vi "ACC_LabVIEW_Connect.vi"(1 "Nomenklatur":string, 3 "return error strings buffer size (Byte)":u32=500, 5 "error in (no error)":errorcluster) -> (14 "DeviceReferenceOut":cluster{"ID":u32}, 19 "error out":errorcluster)   [LabVIEW 2014, in "ACC_LabVIEW.lvlib"]
doc: "Perform a \"read\" inside the GSI - accelerator control system."
uses:
  ACC_LabVIEW.lvlib
  lib/ACC_Interface_Wrapper.dll
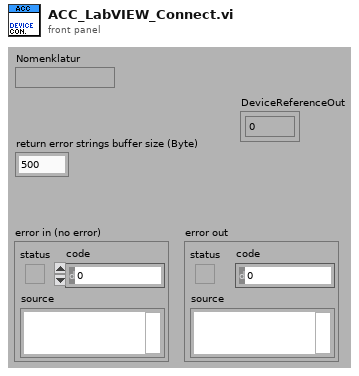
[diagram p1: front panel]
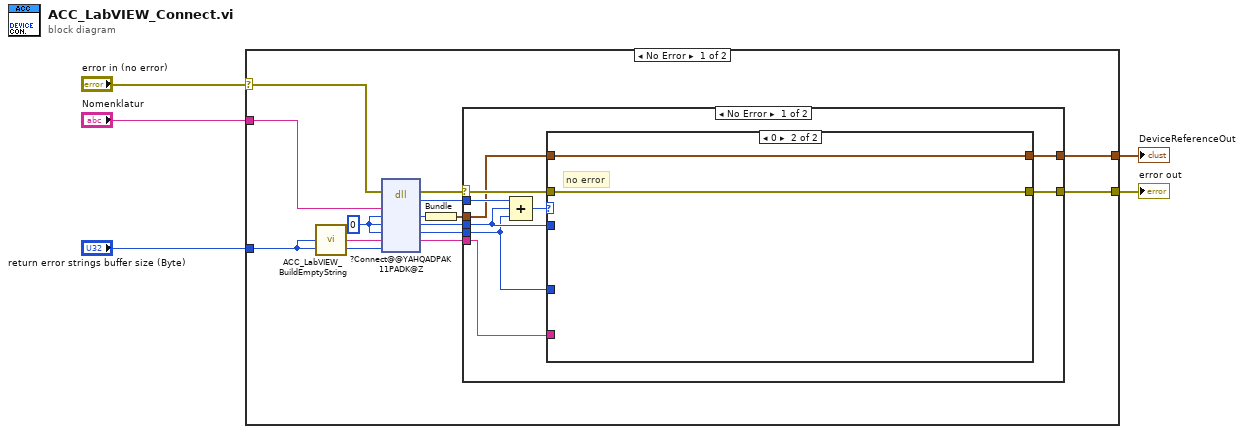
[diagram p0: block diagram]
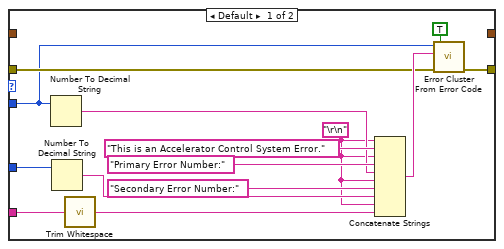
[diagram p2: hidden frame]
diagram:
  n1 = case shown="No Error" "error in (no error)" {
    selector: "error in (no error)" -> [w17 w46]
    tunnel: "Nomenklatur" -> [w18 _]
    tunnel: "return error strings buffer size (Byte)" -> [w15 _]
    tunnel: [w19 w46] -> w3
    tunnel: [w8 _] -> w1
    frame No Error {
      w9 = u32 0 ("no input, only output")
      n2 = call "ACC_LabVIEW_BuildEmptyString.vi"("Length"=w15) -> ("String"=w16:string)
      n3 = dll-call lib="D:/Git/CS-framework/CSinstr.lib/ACC_LabVIEW_Interface/lib/ACC_Interface_Wrapper.dll" fn="?Connect@@YAHQADPAK11PADK@Z"(error in=w17, "LV_nomenklatur"=w18, "DeviceHandle"=w9, "ErrPrimStat"=w9, "ErrSecStat"=w9, "ErrorMSG"=w16, "ErrorMSG_Size"=w15) -> (error out=w14:errorcluster, "ErrorPrimState"=w13:i32, "DeviceHandle"=w7:u32, "ErrPrimStat"=w11:u32, "ErrSecStat"=w10:u32, "ErrorMSG"=w12:string)  [unwired: 4 in, 1 out]
      n4 = Bundle("DeviceHandle"=w7) -> (w6:cluster{"DeviceHandle":u32})  [unwired: 1 in]
      n5 = case shown="No Error" w14 {
        selector: w14 -> [w26 w45]
        tunnel: w13 -> [w28 _]
        tunnel: [w23 w45] -> w19
        tunnel: w12 -> [w22 _]
        tunnel: w11 -> [w25 _]
        tunnel: w10 -> [w24 _]
        tunnel: w6 -> [w21 _]
        tunnel: [w20 _] -> w8
        frame No Error {
          n6 = Compound Arithmetic op=ADD(w28, w25, w24) -> (w27:u32)
          n7 = case shown="0" w27 {
            tunnel: w26 -> [w32 w44]
            tunnel: w25 -> [w30 _]
            tunnel: w24 -> [w42 _]
            tunnel: [w31 w44] -> w23
            tunnel: w22 -> [w36 _]
            tunnel: w21 -> [_ w43]
            tunnel: [_ w43] -> w20
            frame Default {
              w34 = "\r\n"
              n8 = Number To Decimal String(number=w30) -> (decimal integer string=w39:string)  [unwired: 1 in]
              n9 = Number To Decimal String(number=w42) -> (decimal integer string=w37:string)  [unwired: 1 in]
              n10 = call <vilib>:"Trim Whitespace.vi"("string"=w36) -> ("trimmed string"=w35:string)  [unwired: 1 in]
              n11 = Concatenate Strings(w34, "This is an Accelerator Control System Error.", w34, "Primary Error Number:", w39, w34, "Secondary Error Number:", w37, w34, w35) -> (w33:string)
              n12 = call <vilib>:"Error Cluster From Error Code.vi"("show call chain? (False)"=TRUE, "error in (no error)"=w32, "error message (\"\")"=w33, "error code (0)"=w30) -> ("error out"=w31:errorcluster)  [unwired: 5 in]
            }
            frame 0 {
              # "no error"
            }
          }
        }
        frame Error {
        }
      }
    }
    frame Error {
    }
  }
  "error out" <- w3
  "DeviceReferenceOut" <- w1
